vi "GPS Save waypoint list.vi"() -> ()   [LabVIEW 2009]
uses:
  TypeDefs/Sensor TypeDefs/GPS Data.ctl
panel:
  out "List of GPS waypoints":T1[](array[typedef]) {"Longitude" format="%#_14g"; "Latitude" format="%#_14g"}
  in  "stop":bool
  in  "Point Entered":bool
  in  "Latitude Point (degrees)":dbl format="%#_9g"
  in  "Longitude Point (degrees)":dbl format="%#_9g"
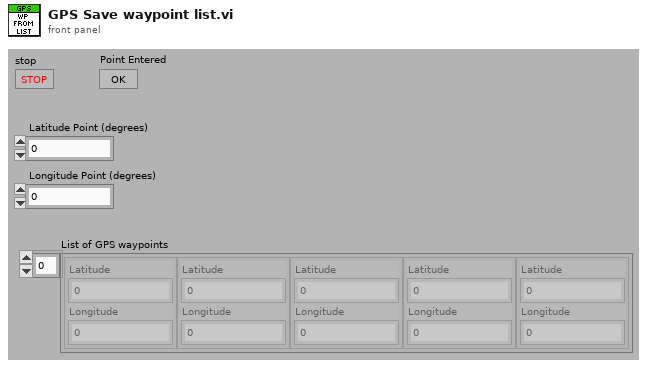
[diagram p1: front panel]
types:
  T1 = typedef "GPS Data.ctl" = cluster{"Latitude":dbl, "Longitude":dbl}
  T2 = enum16{"open", "replace", "create", "open or create", "replace or create", "replace or create with confirmation"}
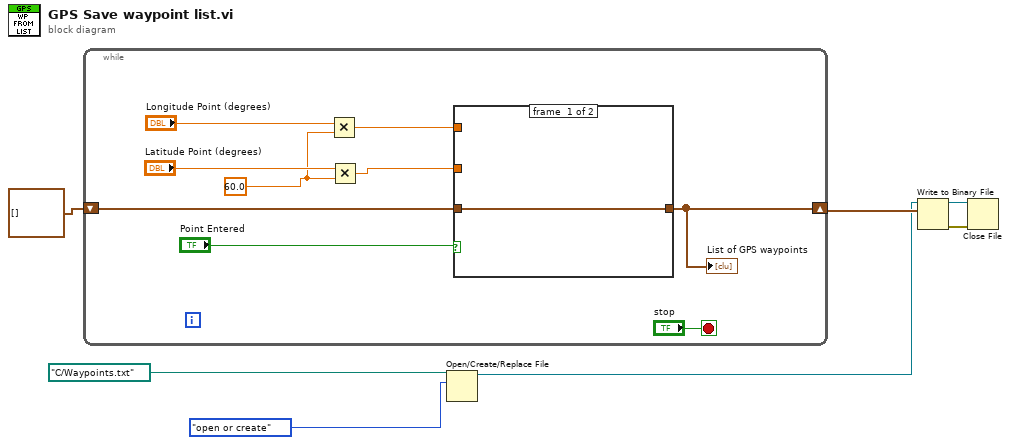
[diagram p0: block diagram]
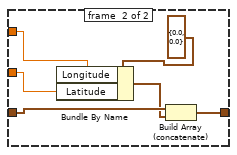
[diagram p2: hidden frame]
diagram:
  n1 = while {
    shift-right: [w12] -> w6
    shift-left: T1[] [] -> [w14]
    stop <- "stop" stop-if-true
    w8 = 60.0 ("y")
    n2 = Multiply(x="Longitude Point (degrees)", y=w8) -> (x*y=w10:dbl)
    n3 = Multiply(x="Latitude Point (degrees)", y=w8) -> (x*y=w9:dbl)
    n4 = case shown="True" "Point Entered" {
      tunnel: w10 -> [_ w23]
      tunnel: w9 -> [_ w22]
      tunnel: [w17 w19] -> w12
      tunnel: w14 -> [w17 w21]
      frame #0 {
      }
      frame #1 {
        n5 = Bundle By Name(cluster=T1 {"Latitude"=0.0, "Longitude"=0.0} ("GPS Point"), "Longitude"=w23, "Latitude"=w22) -> (w20:T1)
        n6 = Build Array (concatenate)(w21, w20) -> (w19:T1[])
      }
    }
    "List of GPS waypoints" <- w12
  }
  n7 = Open/Create/Replace File(file path (use dialog)=path "C:/Waypoints.txt", operation (0:open)=T2."open or create") -> (refnum out=w4:refnum<file>)  [unwired: 4 in, 2 out]
  n8 = Write to Binary File(file (use dialog)=w4, data=w6) -> (refnum out=w2:refnum<file>, error out=w3:errorcluster)  [unwired: 4 in, 1 out]
  n9 = Close File(refnum=w2, error in=w3) -> ()  [unwired: 2 out]
